vi "rs3 export import color Correction.vi"(0 "error in (no error)":errorcluster, 4 "Load/save":enum16{"Load", "Save"}(ring), 5 "STColorCorrection in":T1={"colorCorrection 1"=0.54785156, "colorCorrection 2"=0.32910156, "colorCorrection 3"=0.8222656, "colorCorrection 4"=0.109375, "colorCorrection 5"=-0.40527344, "colorCorrection 6"=-1.5253906, "colorCorrection 7"=0.95703125, "colorCorrection 8"=0.89160156, "colorCorrection 9"=0.7675781, "colorCorrection 10"=-0.4794922, "colorCorrection 11"=0.047851562, "colorCorrection 12"=-0.2705078} {"colorCorrection 1" format="%_4g"}, 6 "file (use dialog)":path) -> (1 "NewJSON":string, 2 "STColorCorrection out":T1={"colorCorrection 1"=0.54785156, "colorCorrection 2"=0.32910156, "colorCorrection 3"=0.8222656, "colorCorrection 4"=0.109375, "colorCorrection 5"=-0.40527344, "colorCorrection 6"=-1.5253906, "colorCorrection 7"=0.95703125, "colorCorrection 8"=0.89160156, "colorCorrection 9"=0.7675781, "colorCorrection 10"=-0.4794922, "colorCorrection 11"=0.047851562, "colorCorrection 12"=-0.2705078} {"colorCorrection 1" format="%_4g"}, 3 "error out":errorcluster={"status"=TRUE, "code"=1430, "source"="Write to Text File in RS2_WriteDepthPreference2.vi<APPEND>\n"})   [LabVIEW 2017, in "libRealSense3.lvlib"]
uses:
  libRealSense3.lvlib
panel:
  # "RS3 Export Color Correction to JSON"
  # "{\n    \"param-censususize\": 9,\n    \"param-censusvsize\": 9,\n    \"param-disableraucolor\": 0,\n    \"param-disablesadcolor\": 0,\n    \"param-disablesadnormalize\": 0,\n    \"param-disablesloleftcolor\": 0,\n    \"param-disableslorightcolor\": 0,\n    \"param-lambdaad\": 800,\n    \"param-lambdacensus\": 26,\n    \"param-leftrightthreshold\": 24,\n    \"param-maxscorethreshb\": 2047,\n    \"param-medianthreshold\": 500,\n    \"param-minscorethresha\": 1,\n    \"param-neighborthresh\": 7,\n    \"param-raumine\": 1,\n    \"param-rauminn\": 1,\n    \"param-rauminnssum\": 3,\n    \"param-raumins\": 1,\n    \"param-rauminw\": 1,\n    \"param-rauminwesum\": 3,\n    \"param-regioncolorthresholdb\": 0.05,\n    \"param-regioncolorthresholdg\": 0.05,\n    \"param-regioncolorthresholdr\": 0.05,\n    \"param-regionshrinku\": 3,\n    \"param-regionshrinkv\": 1,\n    \"param-regionspatialthresholdu\": 7,\n    \"param-regionspatialthresholdv\": 3,\n    \"param-robbinsmonrodecrement\": 10,\n    \"param-robbinsmonroincrement\": 10,\n    \"param-rsmdiffthreshold\": 4.0,\n    \"param-rsmrauslodiffthreshold\": 1.0,\n    \"param-rsmremovethreshold\": 0.3,\n    \"param-scanlineedgetaub\": 72,\n    \"param-scanlineedgetaug\": 72,\n    \"param-scanlineedgetaur\": 72,\n    \"param-scanlinep1\": 180,\n    \"param-scanlinep1onediscon\": 90,\n    \"param-scanlinep1twodiscon\": 59,\n    \"param-scanlinep2\": 342,\n    \"param-scanlinep2onediscon\": 171,\n    \"param-scanlinep2twodiscon\": 113,\n    \"param-secondpeakdelta\": 675,\n    \"param-texturecountthresh\": 0,\n    \"param-texturedifferencethresh\": 0,\n    \"param-usersm\": 1\n}"
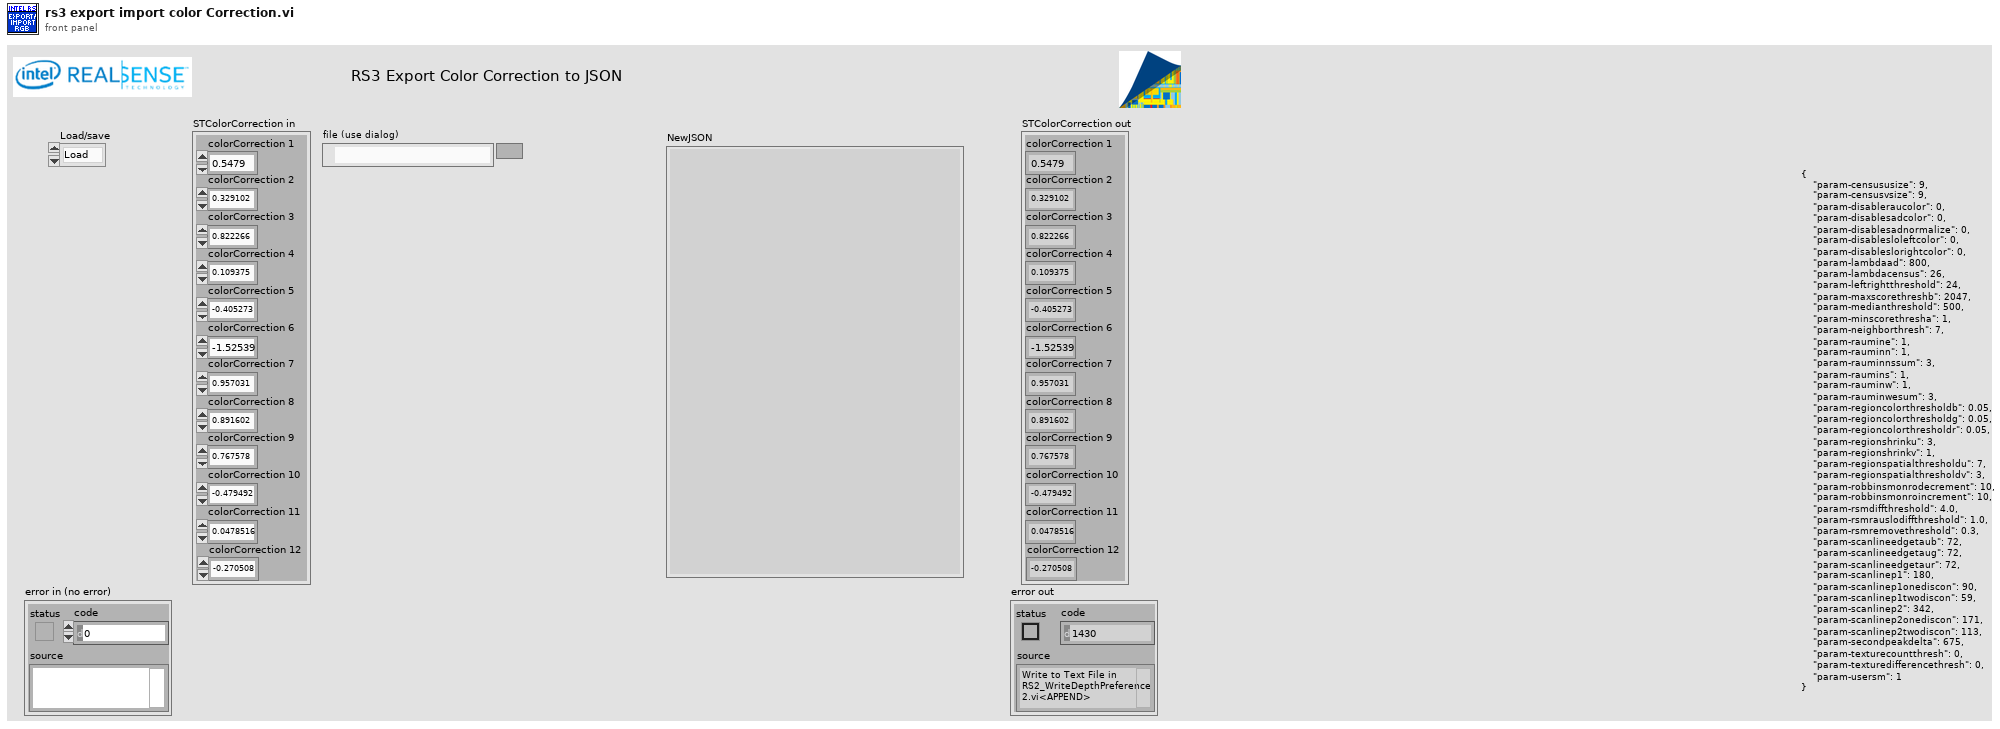
[diagram p1: front panel]
types:
  T1 = cluster{"colorCorrection 1":sgl, "colorCorrection 2":sgl, "colorCorrection 3":sgl, "colorCorrection 4":sgl, "colorCorrection 5":sgl, "colorCorrection 6":sgl, "colorCorrection 7":sgl, "colorCorrection 8":sgl, "colorCorrection 9":sgl, "colorCorrection 10":sgl, "colorCorrection 11":sgl, "colorCorrection 12":sgl}
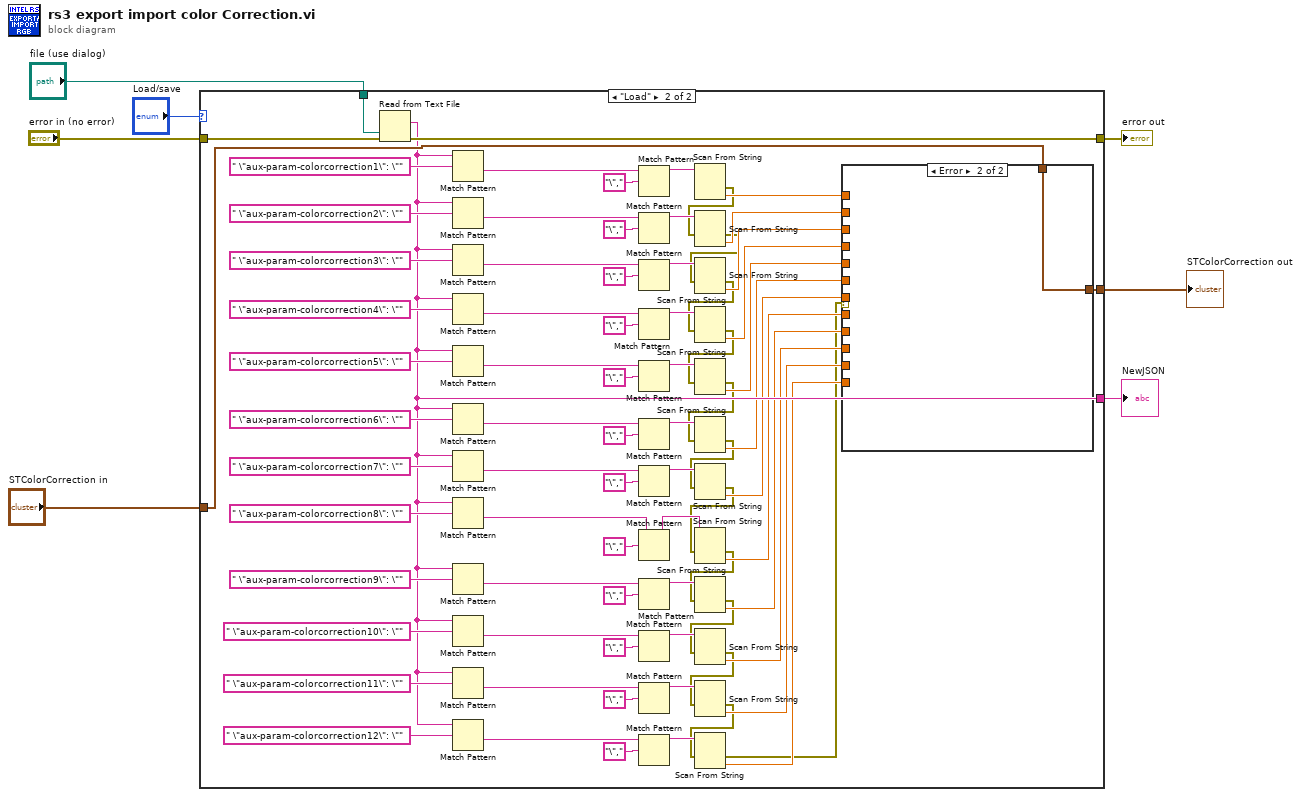
[diagram p0: block diagram]
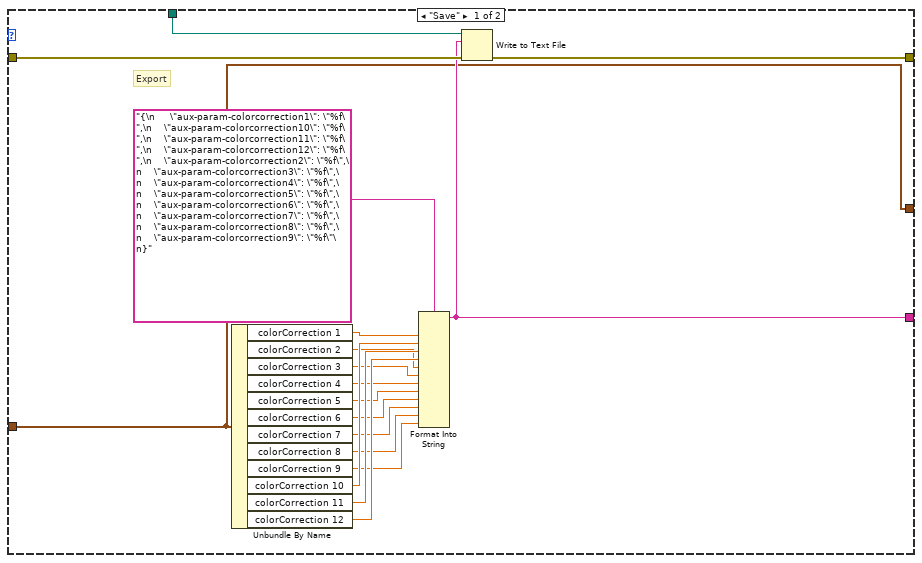
[diagram p2: hidden frame]
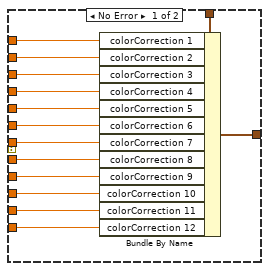
[diagram p3: hidden frame]
diagram:
  n1 = case shown="\"Load\"" "Load/save" {
    tunnel: "error in (no error)" -> [w25 w101]
    tunnel: [w24 w100] -> w6
    tunnel: "STColorCorrection in" -> [w9 w103]
    tunnel: [w10 w49] -> w3
    tunnel: [w9 w102] -> w2
    tunnel: "file (use dialog)" -> [w8 w38]
    frame "Save" {
      # "Export"
      n2 = Unbundle By Name(w9) -> ("colorCorrection 1"=w22:sgl, "colorCorrection 2"=w18:sgl, "colorCorrection 3"=w17:sgl, "colorCorrection 4"=w16:sgl, "colorCorrection 5"=w15:sgl, "colorCorrection 6"=w14:sgl, "colorCorrection 7"=w13:sgl, "colorCorrection 8"=w12:sgl, "colorCorrection 9"=w11:sgl, "colorCorrection 10"=w21:sgl, "colorCorrection 11"=w20:sgl, "colorCorrection 12"=w19:sgl)
      n3 = Format Into String(format string="{\n     \"aux-param-colorcorrection1\": \"%f\",\n    \"aux-param-colorcorrection10\": \"%f\",\n    \"aux-param-colorcorrection11\": \"%f\",\n    \"aux-param-colorcorrection12\": \"%f\",\n    \"aux-param-colorcorrection2\": \"%f\",\n    \"aux-param-colorcorrection3\": \"%f\",\n    \"aux-param-colorcorrection4\": \"%f\",\n    \"aux-param-colorcorrection5\": \"%f\",\n    \"aux-param-colorcorrection6\": \"%f\",\n    \"aux-param-colorcorrection7\": \"%f\",\n    \"aux-param-colorcorrection8\": \"%f\",\n    \"aux-param-colorcorrection9\": \"%f\"\n}" ("regular expression"), w22, w21, w20, w19, w18, w17, w16, w15, w14, w13, w12, w11) -> (resulting string=w10:string)  [unwired: 2 in, 1 out]
      n4 = Write to Text File(file (use dialog)=w8, text=w10, error in=w25) -> (error out=w24:errorcluster)  [unwired: 1 in, 2 out]
    }
    frame "Load" {
      n5 = Read from Text File(file (use dialog)=w38, error in=w101) -> (text=w49:string, error out=w100:errorcluster)  [unwired: 2 in, 2 out]
      n6 = Match Pattern(string=w49, regular expression=" \"aux-param-colorcorrection1\": \"" ("string")) -> (after substring=w98:string)  [unwired: 1 in, 3 out]
      n7 = Match Pattern(string=w49, regular expression=" \"aux-param-colorcorrection2\": \"" ("string")) -> (after substring=w92:string)  [unwired: 1 in, 3 out]
      n8 = Match Pattern(string=w49, regular expression=" \"aux-param-colorcorrection3\": \"" ("string")) -> (after substring=w89:string)  [unwired: 1 in, 3 out]
      n9 = Match Pattern(string=w49, regular expression=" \"aux-param-colorcorrection4\": \"" ("string")) -> (after substring=w84:string)  [unwired: 1 in, 3 out]
      n10 = Match Pattern(string=w49, regular expression=" \"aux-param-colorcorrection5\": \"" ("string")) -> (after substring=w81:string)  [unwired: 1 in, 3 out]
      n11 = Match Pattern(string=w49, regular expression=" \"aux-param-colorcorrection6\": \"" ("string")) -> (after substring=w76:string)  [unwired: 1 in, 3 out]
      n12 = Match Pattern(string=w49, regular expression=" \"aux-param-colorcorrection7\": \"" ("string")) -> (after substring=w73:string)  [unwired: 1 in, 3 out]
      n13 = Match Pattern(string=w49, regular expression=" \"aux-param-colorcorrection8\": \"" ("string")) -> (after substring=w68:string)  [unwired: 1 in, 3 out]
      n14 = Match Pattern(string=w49, regular expression=" \"aux-param-colorcorrection9\": \"" ("string")) -> (after substring=w65:string)  [unwired: 1 in, 3 out]
      n15 = Match Pattern(string=w49, regular expression=" \"aux-param-colorcorrection10\": \"" ("string")) -> (after substring=w60:string)  [unwired: 1 in, 3 out]
      n16 = Match Pattern(string=w49, regular expression=" \"aux-param-colorcorrection11\": \"" ("string")) -> (after substring=w56:string)  [unwired: 1 in, 3 out]
      n17 = Match Pattern(string=w49, regular expression=" \"aux-param-colorcorrection12\": \"" ("string")) -> (after substring=w51:string)  [unwired: 1 in, 3 out]
      n18 = Match Pattern(string=w98, regular expression="\",") -> (before substring=w96:string)  [unwired: 1 in, 3 out]
      n19 = Match Pattern(string=w92, regular expression="\",") -> (before substring=w94:string)  [unwired: 1 in, 3 out]
      n20 = Match Pattern(string=w89, regular expression="\",") -> (before substring=w87:string)  [unwired: 1 in, 3 out]
      n21 = Match Pattern(string=w84, regular expression="\",") -> (before substring=w86:string)  [unwired: 1 in, 3 out]
      n22 = Match Pattern(string=w81, regular expression="\",") -> (before substring=w79:string)  [unwired: 1 in, 3 out]
      n23 = Match Pattern(string=w76, regular expression="\",") -> (before substring=w78:string)  [unwired: 1 in, 3 out]
      n24 = Match Pattern(string=w73, regular expression="\",") -> (before substring=w71:string)  [unwired: 1 in, 3 out]
      n25 = Match Pattern(string=w68, regular expression="\",") -> (before substring=w70:string)  [unwired: 1 in, 3 out]
      n26 = Match Pattern(string=w65, regular expression="\",") -> (before substring=w63:string)  [unwired: 1 in, 3 out]
      n27 = Match Pattern(string=w60, regular expression="\",") -> (before substring=w62:string)  [unwired: 1 in, 3 out]
      n28 = Match Pattern(string=w56, regular expression="\",") -> (before substring=w54:string)  [unwired: 1 in, 3 out]
      n29 = Match Pattern(string=w51, regular expression="\",") -> (before substring=w53:string)  [unwired: 1 in, 3 out]
      n30 = Scan From String(input string=w96) -> (error out=w37:errorcluster, output 1=w95:dbl)  [unwired: 4 in, 2 out]
      n31 = Scan From String(input string=w94, error in=w37) -> (error out=w36:errorcluster, output 1=w58:dbl)  [unwired: 3 in, 2 out]
      n32 = Scan From String(input string=w87, error in=w36) -> (error out=w35:errorcluster, output 1=w48:dbl)  [unwired: 3 in, 2 out]
      n33 = Scan From String(input string=w86, error in=w35) -> (error out=w34:errorcluster, output 1=w47:dbl)  [unwired: 3 in, 2 out]
      n34 = Scan From String(input string=w79, error in=w34) -> (error out=w33:errorcluster, output 1=w46:dbl)  [unwired: 3 in, 2 out]
      n35 = Scan From String(input string=w78, error in=w33) -> (error out=w32:errorcluster, output 1=w45:dbl)  [unwired: 3 in, 2 out]
      n36 = Scan From String(input string=w71, error in=w32) -> (error out=w31:errorcluster, output 1=w44:dbl)  [unwired: 3 in, 2 out]
      n37 = Scan From String(input string=w70, error in=w31) -> (error out=w30:errorcluster, output 1=w43:dbl)  [unwired: 3 in, 2 out]
      n38 = Scan From String(input string=w63, error in=w30) -> (error out=w29:errorcluster, output 1=w42:dbl)  [unwired: 3 in, 2 out]
      n39 = Scan From String(input string=w62, error in=w29) -> (error out=w28:errorcluster, output 1=w41:dbl)  [unwired: 3 in, 2 out]
      n40 = Scan From String(input string=w54, error in=w28) -> (error out=w27:errorcluster, output 1=w40:dbl)  [unwired: 3 in, 2 out]
      n41 = Scan From String(input string=w53, error in=w27) -> (error out=w26:errorcluster, output 1=w39:dbl)  [unwired: 3 in, 2 out]
      n42 = case shown="Error" w26 {
        tunnel: w103 -> [w117 w118]
        tunnel: [w116 w118] -> w102
        tunnel: w95 -> [w115 _]
        tunnel: w58 -> [w114 _]
        tunnel: w48 -> [w113 _]
        tunnel: w47 -> [w112 _]
        tunnel: w46 -> [w111 _]
        tunnel: w45 -> [w110 _]
        tunnel: w44 -> [w109 _]
        tunnel: w43 -> [w108 _]
        tunnel: w42 -> [w107 _]
        tunnel: w41 -> [w106 _]
        tunnel: w40 -> [w105 _]
        tunnel: w39 -> [w104 _]
        frame No Error {
          n43 = Bundle By Name(cluster=w117, "colorCorrection 1"=w115, "colorCorrection 2"=w114, "colorCorrection 3"=w113, "colorCorrection 4"=w112, "colorCorrection 5"=w111, "colorCorrection 6"=w110, "colorCorrection 7"=w109, "colorCorrection 8"=w108, "colorCorrection 9"=w107, "colorCorrection 10"=w106, "colorCorrection 11"=w105, "colorCorrection 12"=w104) -> (w116:T1)
        }
        frame Error {
        }
      }
    }
  }
  "error out" <- w6
  "STColorCorrection out" <- w2
  "NewJSON" <- w3
